vi "SetAmplitudeRange.vi"(7 "reference level offset":dbl, 8 "error in (no error)":errorcluster, 9 "Attenuation":dbl format="%#_13g", 10 "Ref Level":dbl format="%#_13g", 11 "KeysightN9020B in":refnum<class "KeysightN9020B.lvclass">) -> (0 "error out":errorcluster, 3 "KeysightN9020B out":refnum<class "KeysightN9020B.lvclass">)   [LabVIEW 2023, in "KeysightN9020B.lvlib" / "KeysightN9020B.lvclass"]
uses:
  KeysightN9020B.lvclass
  <vilib>/ActorFramework/Actor/Actor.lvclass/Actor.ctl
  KeysightN9020B.lvclass/KeysightN9020B.ctl
  <vilib>/ActorFramework/Message Enqueuer/Message Enqueuer.lvclass/Message Enqueuer.ctl
  <vilib>/ActorFramework/Message Enqueuer/Enqueue.vi
  Interfaces/AbstractInstrumentClasses/SpectrumAnalyzer_LV/SpectrumAnalyzerComm Messages/SpectrumConfigDone Msg/SpectrumConfigDone Msg.lvclass
  <vilib>/ActorFramework/Message Priority Queue/Priority Enqueue.vi
  <instrlib>/Keysight XSAn/Keysight XSAn.lvlib
  <vilib>/ActorFramework/Actor/Actor.lvclass
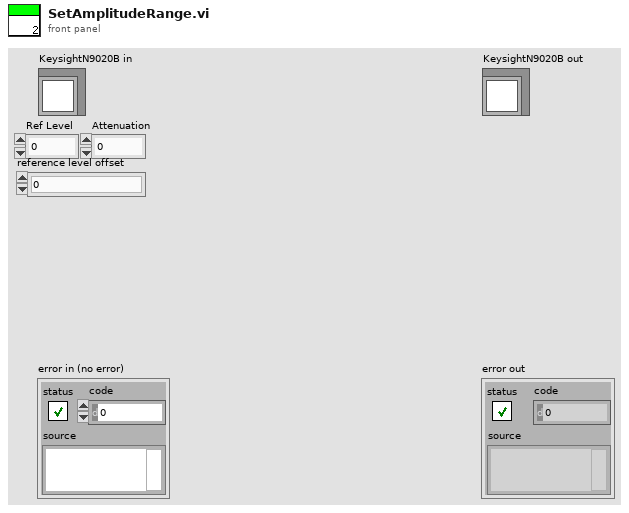
[diagram p1: front panel]
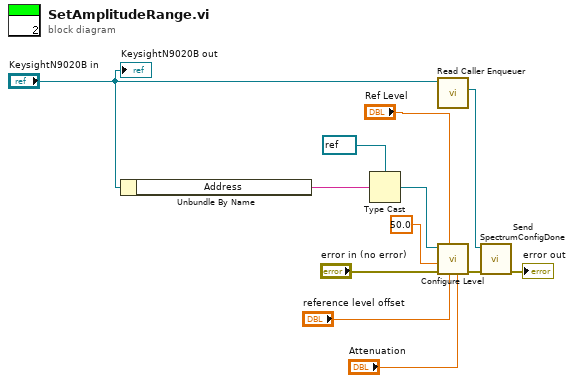
[diagram p0: block diagram]
diagram:
  n1 = Unbundle By Name("KeysightN9020B in") -> ("Address"=w7:string)
  n2 = Type Cast(type=refnum<k15> refnum ("instrument handle"), x=w7) -> (*(type *) &x=w5:refnum<k15>)
  n3 = call <vilib>:"Read Caller Enqueuer.vi"("Actor"="KeysightN9020B in") -> ("Caller Enqueuer"=w4:refnum<class "Message Enqueuer.lvclass">)  [unwired: 10 in]
  n4 = call <instrlib>:"Configure Level.vi"("attenuation"="Attenuation", "reference level offset"="reference level offset", "reference level"="Ref Level", "error in (no error)"="error in (no error)", "input impedance"=50.0, "instrument handle"=w5) -> ("error out"=w3:errorcluster)  [unwired: 4 in, 1 out]
  n5 = call "Send SpectrumConfigDone.vi"("error in (no error)"=w3, "Message Enqueuer"=w4) -> ("error out"=→"error out":errorcluster)  [unwired: 8 in, 1 out]
  "KeysightN9020B out" <- "KeysightN9020B in"
